vi "Max_Totzeit.vi"(6 "Totzeit":dbl, 8 "error in (no error)":errorcluster, 9 "Reset":bool, 10 "Enable":bool=TRUE, 11 "Signals":dynamicdata(graph)) -> (0 "error out":errorcluster, 3 "Delayed Signals":dynamicdata(graph))   [LabVIEW 2015]
doc: "Stores data from previous iterations of a loop and passes the data after the specified number of iterations occur.\n--------------------\n\nThis Express VI is configured as follows:\n\nHistory Size: 1"
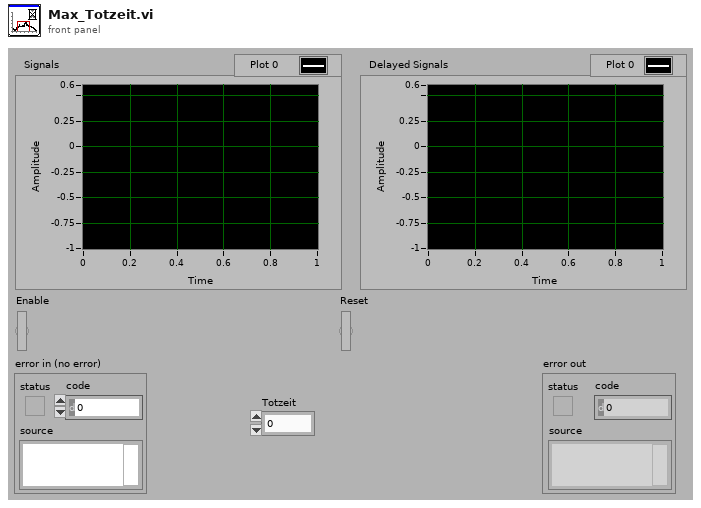
[diagram p1: front panel]
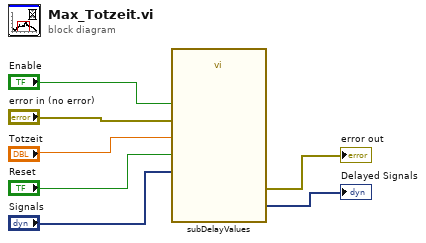
[diagram p0: block diagram]
diagram:
  n1 = call <vilib>:"subDelayValues.vi"("History Size"="Totzeit", "error in (no error)"="error in (no error)", "Reset"="Reset", "Enable"="Enable", "Signals"="Signals") -> ("error out"=→"error out":errorcluster, "Result"=→"Delayed Signals":dynamicdata)  [unwired: 5 in]
